vi "ApplyVIPC.vi"   [LabVIEW 2021]
uses:
  <vilib>/Wiresmith Technology/G CLI/CLI Class/CLI.lvclass
  <vilib>/JKI/VIPM API/VIPM API_vipm_api.lvlib
types:
  T1 = enum32{"Invalid", "Standard", "Closed", "Hidden", "Minimized", "Maximized"}
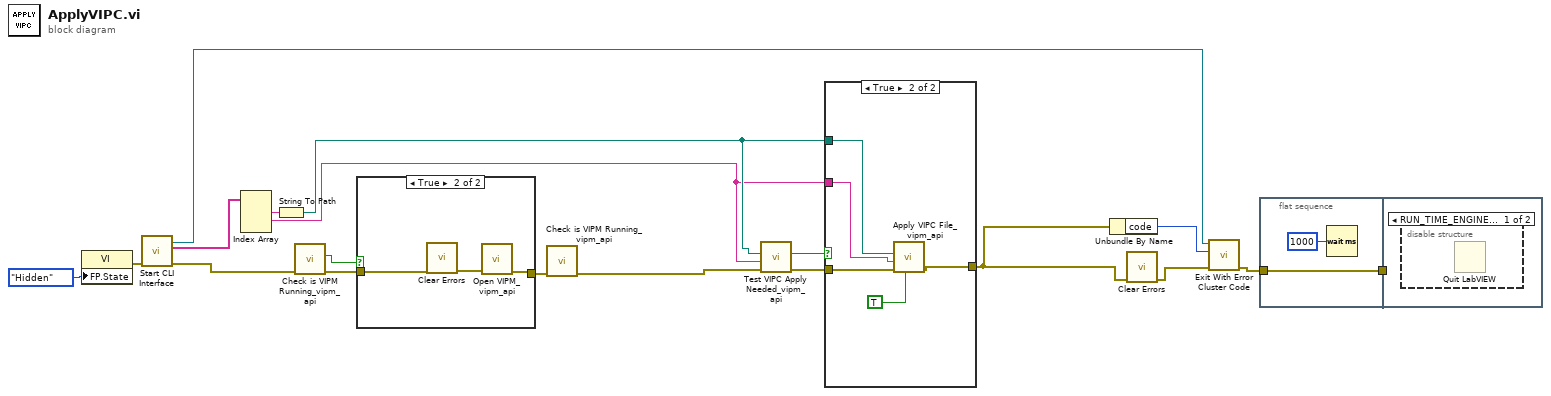
[diagram p0: block diagram]
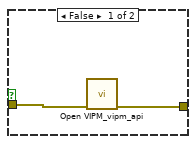
[diagram p2: hidden frame]
diagram:
  n1 = property class="VI"("FP.State"=T1."Hidden" ("Front Panel Window:State")) -> (error out=w18:errorcluster)  [unwired: 2 in, 1 out]
  n2 = call <vilib>:"Start CLI Interface.vi"("error in (no error)"=w18) -> ("error out"=w3:errorcluster, "Custom Parameters"=w16:string[], "CLI out"=w17:refnum<class "CLI.lvclass">)  [unwired: 7 in, 1 out]
  n3 = Index Array(array=w16) -> (element #1=w13:string, element #2=w9:string)  [unwired: 3 in, 1 out]
  n4 = String To Path(string=w13) -> (path=w10:path)
  n5 = call <vilib>:"Check is VIPM Running_vipm_api.vi"("error in (no error)"=w3) -> ("error out"=w8:errorcluster, "is Running"=w7:bool)  [unwired: 9 in]
  n6 = case shown="True" w7 {
    tunnel: w8 -> [w21 w22]
    tunnel: [w20 w23] -> w6
    frame False {
      n7 = call <vilib>:"Open VIPM_vipm_api.vi"("error in (no error)"=w21) -> ("error out"=w20:errorcluster)  [unwired: 10 in]
    }
    frame True {
      n8 = call <vilib>:"Clear Errors.vi"("error in (no error)"=w22) -> ("error out"=w24:errorcluster)  [unwired: 5 in, 1 out]
      n9 = call <vilib>:"Open VIPM_vipm_api.vi"("error in (no error)"=w24) -> ("error out"=w23:errorcluster)  [unwired: 10 in]
    }
  }
  n10 = call <vilib>:"Check is VIPM Running_vipm_api.vi"("error in (no error)"=w6) -> ("error out"=w4:errorcluster)  [unwired: 9 in, 1 out]
  n11 = call <vilib>:"Test VIPC Apply Needed_vipm_api.vi"("error in (no error)"=w4, "LabVIEW Version (use vipc version)"=w9, "VIPC File Path"=w10) -> ("error out"=w11:errorcluster, "Need to Apply?"=w12:bool)  [unwired: 6 in, 1 out]
  n12 = case shown="True" w12 {
    tunnel: w11 -> [w25 w29]
    tunnel: [w25 w28] -> w5
    tunnel: w10 -> [_ w27]
    tunnel: w9 -> [_ w26]
    frame False {
    }
    frame True {
      n13 = call <vilib>:"Apply VIPC File_vipm_api.vi"("quiet? (T)"=TRUE, "error in (no error)"=w29, "LabVIEW Version"=w26, "VIPC File"=w27) -> ("error out"=w28:errorcluster)  [unwired: 7 in]
    }
  }
  n14 = Unbundle By Name(w5) -> ("code"=w2:i32)
  n15 = call <vilib>:"Clear Errors.vi"("error in (no error)"=w5) -> ("error out"=w1:errorcluster)  [unwired: 5 in, 1 out]
  n16 = call <vilib>:"Exit With Error Cluster Code.vi"("error in (no error)"=w1, "No Error Code (0)"=w2, "CLI in"=w17) -> ("error out"=w14:errorcluster)  [unwired: 8 in]
  n17 = flat-sequence {
    tunnel: w14 -> [w32]
    tunnel: [w32] -> w15
    tunnel: w15 -> [_]
    frame #0 {
      n18 = Wait (ms)(milliseconds to wait=u32 1000) -> ()  [unwired: 1 out]
    }
    frame #1 {
      n19 = disable-structure shown="RUN_TIME_ENGINE==True" {
        frame condition #0 {
          n20 = Quit LabVIEW() -> ()  [unwired: 1 in]
        }
        frame condition #1 (active) {
        }
      }
    }
  }
